vi "Change Panel State.vi"(6 "Action":T1, 7 "Connection Name":string, 8 "error in (no error)":errorcluster, 10 "Module ID":i32=-1) -> (0 "error out":errorcluster)   [LabVIEW 2017]
uses:
  Panel Actions.ctl
  Libraries/SSH/SSH.lvlib
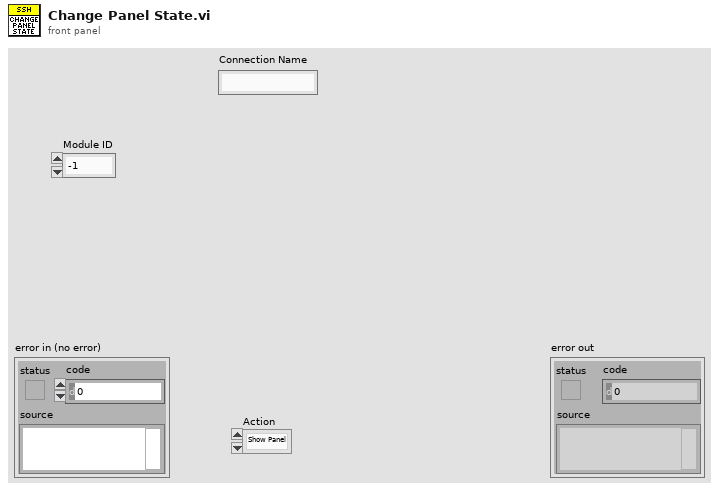
[diagram p1: front panel]
types:
  T1 = typedef "Panel Actions.ctl" = enum16{"Show Panel", "Hide Panel"}
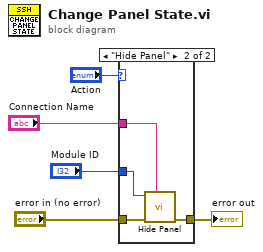
[diagram p0: block diagram]
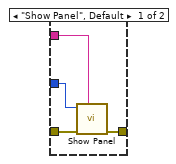
[diagram p2: hidden frame]
diagram:
  n1 = case shown="\"Hide Panel\"" "Action" {
    tunnel: "Connection Name" -> [w9 w10]
    tunnel: "error in (no error)" -> [w8 w13]
    tunnel: "Module ID" -> [w7 w11]
    tunnel: [w6 w12] -> w2
    frame "Show Panel", Default {
      n2 = call "Show Panel.vi"("Connection Name"=w9, "error in (no error)"=w8, "Module ID"=w7) -> ("error out"=w6:errorcluster)  [unwired: 8 in]
    }
    frame "Hide Panel" {
      n3 = call "Hide Panel.vi"("Connection Name"=w10, "error in (no error)"=w13, "Module ID"=w11) -> ("error out"=w12:errorcluster)  [unwired: 8 in]
    }
  }
  "error out" <- w2
